vi "Read Math Average Parameters.vi"(0 "VISA resource name":refnum<visa-resource-name>, 11 "error in (no error)":errorcluster) -> (3 "Minimum":dbl, 4 "VISA resource name out":refnum<visa-resource-name>, 6 "Average Value":dbl, 8 "Count":dbl, 10 "Maximum":dbl, 15 "error out":errorcluster)   [LabVIEW 2013, in "DmmPwr Simulator.lvlib"]
doc: "Gets the average math settings from the instrument."
uses:
  <instrlib>/DmmPwr Simulator/DmmPwr Simulator.lvlib
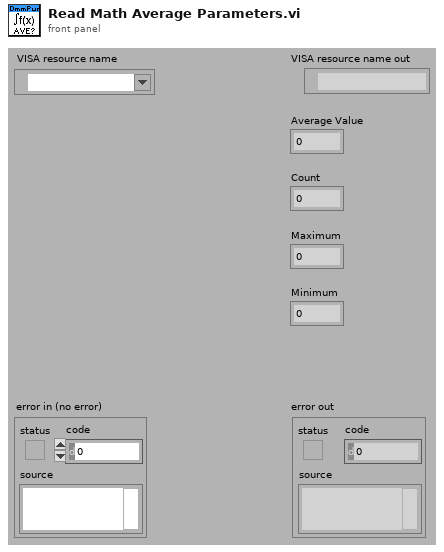
[diagram p1: front panel]
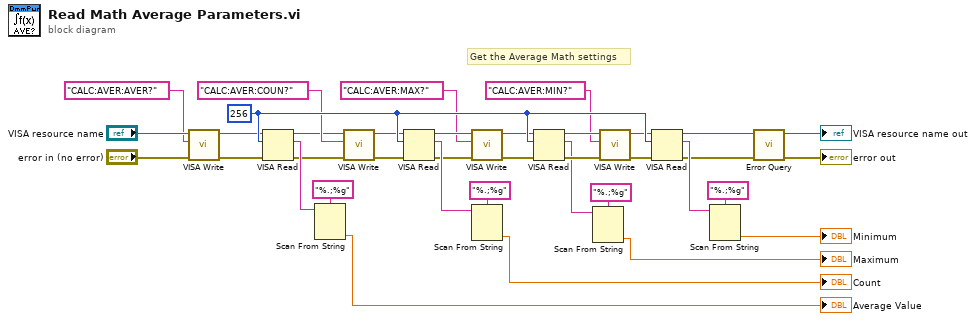
[diagram p0: block diagram]
diagram:
  w34 = u32 256 ("byte count")
  # "Get the Average Math settings"
  n1 = call <instrlib>:"VISA Write.vi"("error in"="error in (no error)", "write buffer"="CALC:AVER:AVER?", "VISA resource name"="VISA resource name") -> ("error out"=w23:errorcluster, "VISA resource name out"=w22:refnum<visa-resource-name>)  [unwired: 6 in, 1 out]
  n2 = VISA Read(VISA resource name=w22, byte count=w34, error in (no error)=w23) -> (VISA resource name out=w16:refnum<visa-resource-name>, read buffer=w37:string, error out=w18:errorcluster)  [unwired: 1 out]
  n3 = Scan From String(format string="%.;%g", input string=w37) -> (output 1=→"Average Value":dbl)  [unwired: 2 in, 4 out]
  n4 = call <instrlib>:"VISA Write.vi"("error in"=w18, "write buffer"="CALC:AVER:COUN?", "VISA resource name"=w16) -> ("error out"=w19:errorcluster, "VISA resource name out"=w20:refnum<visa-resource-name>)  [unwired: 6 in, 1 out]
  n5 = VISA Read(VISA resource name=w20, byte count=w34, error in (no error)=w19) -> (VISA resource name out=w12:refnum<visa-resource-name>, read buffer=w30:string, error out=w15:errorcluster)  [unwired: 1 out]
  n6 = call <instrlib>:"VISA Write.vi"("error in"=w15, "write buffer"="CALC:AVER:MAX?", "VISA resource name"=w12) -> ("error out"=w14:errorcluster, "VISA resource name out"=w13:refnum<visa-resource-name>)  [unwired: 6 in, 1 out]
  n7 = Scan From String(format string="%.;%g", input string=w30) -> (output 1=→"Count":dbl)  [unwired: 2 in, 4 out]
  n8 = VISA Read(VISA resource name=w13, byte count=w34, error in (no error)=w14) -> (VISA resource name out=w9:refnum<visa-resource-name>, read buffer=w7:string, error out=w10:errorcluster)  [unwired: 1 out]
  n9 = Scan From String(format string="%.;%g", input string=w7) -> (output 1=→"Maximum":dbl)  [unwired: 2 in, 4 out]
  n10 = call <instrlib>:"VISA Write.vi"("error in"=w10, "write buffer"="CALC:AVER:MIN?", "VISA resource name"=w9) -> ("error out"=w8:errorcluster, "VISA resource name out"=w5:refnum<visa-resource-name>)  [unwired: 6 in, 1 out]
  n11 = VISA Read(VISA resource name=w5, byte count=w34, error in (no error)=w8) -> (VISA resource name out=w4:refnum<visa-resource-name>, read buffer=w29:string, error out=w3:errorcluster)  [unwired: 1 out]
  n12 = Scan From String(format string="%.;%g", input string=w29) -> (output 1=→"Minimum":dbl)  [unwired: 2 in, 4 out]
  n13 = call <instrlib>:"Error Query.vi"("error in (no error)"=w3, "VISA resource name"=w4) -> ("error out"=→"error out":errorcluster, "VISA resource name out"=→"VISA resource name out":refnum<visa-resource-name>)  [unwired: 6 in, 2 out]
